vi "DB insert array data（Feedback).vi"(5 "Condtion":string, 7 "Data":string[](array[string]), 8 "error in (no error)":errorcluster caption="错误输入（无错误）", 9 "index":i32, 10 "table":string, 11 "Connncet State":T1) -> (0 "error out":errorcluster caption="错误输出", 1 "state":bool, 3 "Connncet State out":T1)   [LabVIEW 2014]
uses:
  <vilib>/addons/database/NI_Database_API.lvlib
  Ctr/Constr.ctl
  <vilib>/addons/database/Connection.llb/Conn ObjectReference.ctl
  Ctr/Conneect State.ctl
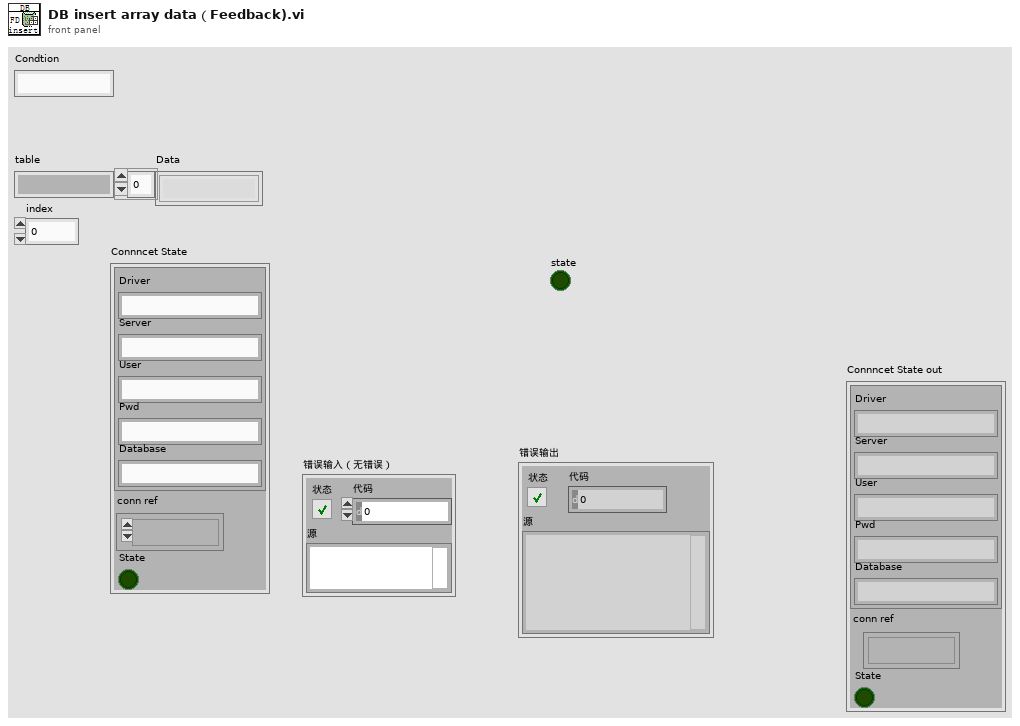
[diagram p1: front panel]
types:
  T1 = typedef "Conneect State.ctl" = cluster{"Constr":T2, "conn ref":T3, "State":bool}
  T2 = typedef "Constr.ctl" = cluster{"Driver":string, "Server":string, "User":string, "Pwd":string, "Database":string}
  T3 = typedef "NI_Database_API.lvlib/Conn ObjectReference.ctl" = refnum<k1>
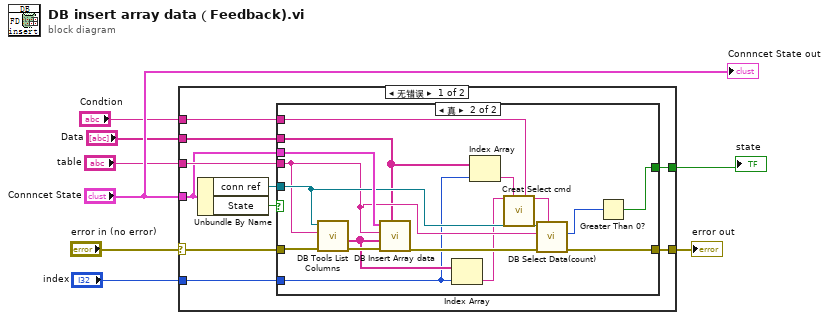
[diagram p0: block diagram]
diagram:
  n1 = case shown="无错误" "error in (no error)" {
    selector: "error in (no error)" -> [w17 w36]
    tunnel: "Connncet State" -> [w14 _]
    tunnel: "table" -> [w15 _]
    tunnel: "Data" -> [w13 _]
    tunnel: "index" -> [w12 _]
    tunnel: [w11 w36] -> w3
    tunnel: [w10 _] -> w2
    tunnel: "Condtion" -> [w9 _]
    frame No Error {
      n2 = Unbundle By Name(w14) -> ("conn ref"=w16:T3, "State"=w18:bool)
      n3 = case shown="真" w18 {
        tunnel: w17 -> [w19 w35]
        tunnel: w16 -> [_ w31]
        tunnel: w15 -> [_ w30]
        tunnel: w14 -> [_ w33]
        tunnel: w13 -> [_ w27]
        tunnel: w12 -> [_ w26]
        tunnel: [w19 w24] -> w11
        tunnel: [_ w22] -> w10
        tunnel: w9 -> [_ w20]
        frame False {
        }
        frame True {
          n4 = call <vilib>:"DB Tools List Columns.vi"("error in (no error)"=w35, "table"=w30, "connection reference"=w31) -> ("error out"=w34:errorcluster, "columns"=w29:string[])  [unwired: 1 in, 2 out]
          n5 = call "DB Insert Array data.vi"("Dtat"=w27, "error in (no error)"=w34, "columns"=w29, "table"=w30, "Connncet State"=w33) -> ("error out"=w32:errorcluster)  [unwired: 5 in, 1 out]
          n6 = Index Array(array=w29, index=w26) -> (element=w28:string)
          n7 = Index Array(array=w27, index=w26) -> (element=w25:string)
          n8 = call "Creat Select cmd.vi"("Col"=w28, "Code"=w25, "Condtion"=w20) -> ("Str"=w21:string)  [unwired: 11 in, 1 out]
          n9 = call "DB Select Data(count).vi"("condition"=w21, "error in (no error)"=w32, "table"=w30, "connection reference"=w31) -> ("error out"=w24:errorcluster, "Count"=w23:i32)  [unwired: 5 in, 1 out]
          n10 = Greater Than 0?(x=w23) -> (x > 0?=w22:bool)
        }
      }
    }
    frame Error {
    }
  }
  "error out" <- w3
  "state" <- w2
  "Connncet State out" <- "Connncet State"
